vi "Client Message.vi"(8 "error in (no error)":errorcluster, 9 "Context":variant, 10 "Message":string, 11 "TCP Communications in":refnum<class "TCP Communications.lvclass">) -> (0 "error out":errorcluster, 1 "Context out":variant, 3 "TCP Communications out":refnum<class "TCP Communications.lvclass">)   [LabVIEW 2019, in "TCP Communications.lvclass"]
uses:
  TCP Communications.lvclass
  Communications/Communications.lvclass
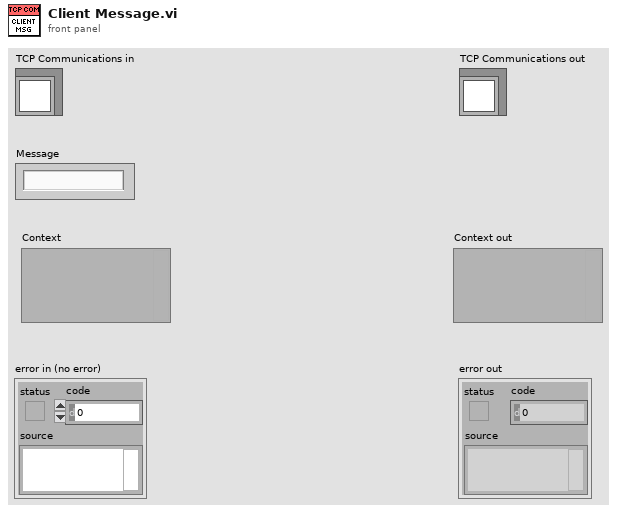
[diagram p1: front panel]
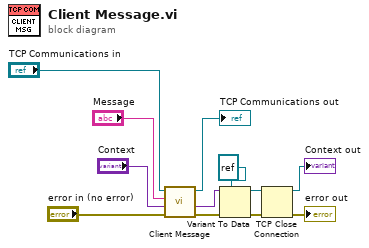
[diagram p0: block diagram]
diagram:
  n1 = call-parent "Client Message.vi"("error in (no error)"="error in (no error)", "Context"="Context", "Message"="Message", "Communications in"="TCP Communications in") -> ("error out"=w3:errorcluster, "Context out"=w2:variant, "Communications out"=→"TCP Communications out":refnum<class "TCP Communications.lvclass">)  [unwired: 5 in]
  n2 = Variant To Data(error in=w3, type=refnum<k5> refnum ("connection ID"), Variant=w2) -> (data=w6:refnum<k5>, error out=w5:errorcluster)
  n3 = TCP Close Connection(connection ID=w6, error in (no error)=w5) -> (connection ID out=→"Context out":refnum<k5>, error out=→"error out":errorcluster)  [unwired: 1 in]
